vi "Source Hi-C Mode.vi"(0 "VISA resource name":refnum<visa-resource-name>, 1 "Set/Query Hi-C Mode":u8(ring) items=["Query", "Set"], 5 "Node In":string, 7 "Channel (Channel A)":u8(ring) items=["Channel A", "Channel B"], 9 "Hi-C Mode Function (Disabled)":u8(ring) items=["Disabled", "Enabled"], 11 "error in (no error)":errorcluster) -> (4 "VISA resource name out":refnum<visa-resource-name>, 6 "Node Out":string, 8 "Hi-C Mode Query Results":string, 15 "error out":errorcluster)   [LabVIEW 2012, in "Keithley 2600 Series.lvlib"]
doc: "This VI can either set the unit into High Capacitance mode or query if the specified channel for High Capacitance mode operation."
uses:
  Keithley 2600 Series.lvlib
panel:
  # "(c) 2009 Keithley Instruments, Inc.  ALL RIGHTS RESERVED."
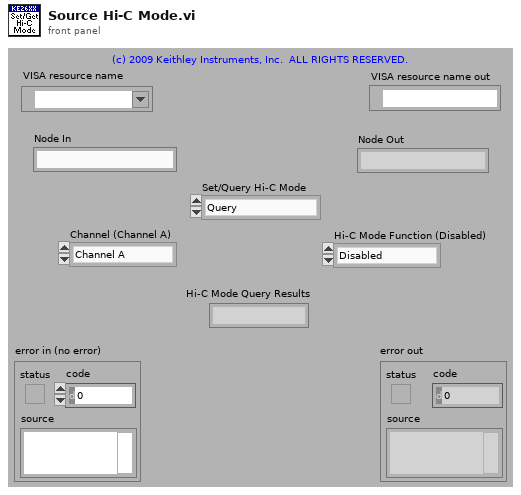
[diagram p1: front panel]
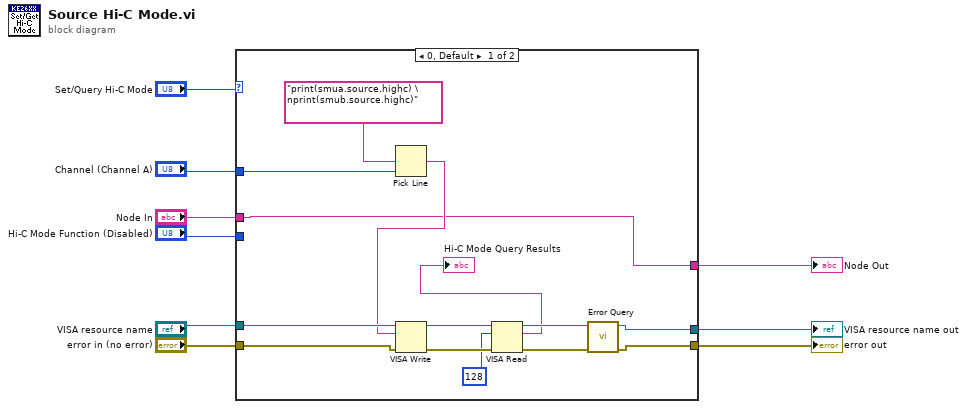
[diagram p0: block diagram]
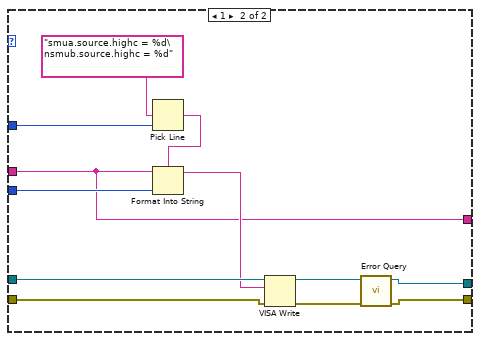
[diagram p2: hidden frame]
diagram:
  n1 = case shown="0, Default" "Set/Query Hi-C Mode" {
    tunnel: [w20 w35] -> w9
    tunnel: [w21 w34] -> w8
    tunnel: "error in (no error)" -> [w17 w31]
    tunnel: "VISA resource name" -> [w16 w30]
    tunnel: "Channel (Channel A)" -> [w14 w28]
    tunnel: "Hi-C Mode Function (Disabled)" -> [_ w26]
    tunnel: "Node In" -> [w11 w24]
    tunnel: [w11 w24] -> w1
    frame 0, Default {
      n2 = Pick Line(multi-line string="print(smua.source.highc) \nprint(smub.source.highc)", line index=w14) -> (output string=w12:string)  [unwired: 1 out]
      n3 = VISA Write(VISA resource name=w16, write buffer=w12, error in (no error)=w17) -> (VISA resource name out=w19:refnum<visa-resource-name>, error out=w18:errorcluster)  [unwired: 1 out]
      n4 = VISA Read(VISA resource name=w19, byte count=128, error in (no error)=w18) -> (VISA resource name out=w23:refnum<visa-resource-name>, read buffer=→"Hi-C Mode Query Results":string, error out=w22:errorcluster)  [unwired: 1 out]
      n5 = call "Error Query.vi"("error in (no error)"=w22, "VISA resource name"=w23) -> ("error out"=w21:errorcluster, "VISA resource name out"=w20:refnum<visa-resource-name>)  [unwired: 8 out]
    }
    frame 1 {
      n6 = Pick Line(multi-line string="smua.source.highc = %d\nsmub.source.highc = %d", line index=w28) -> (output string=w27:string)  [unwired: 1 out]
      n7 = Format Into String(format string=w27, initial string=w24, w26) -> (resulting string=w25:string)  [unwired: 1 in, 1 out]
      n8 = VISA Write(VISA resource name=w30, write buffer=w25, error in (no error)=w31) -> (VISA resource name out=w32:refnum<visa-resource-name>, error out=w33:errorcluster)  [unwired: 1 out]
      n9 = call "Error Query.vi"("error in (no error)"=w33, "VISA resource name"=w32) -> ("error out"=w34:errorcluster, "VISA resource name out"=w35:refnum<visa-resource-name>)  [unwired: 8 out]
    }
  }
  "VISA resource name out" <- w9
  "error out" <- w8
  "Node Out" <- w1
